vi "Assert DB Update Value.vi"() -> ()   [LabVIEW 2015, in "Database.lvclass"]
uses:
  Database.lvclass
panel:
  in  "table":string="钱凌峰ExcuseNote"
  in  "condition":string="Where 姓名= '钱凌峰' and 学号='1110810220' and 日期='2016/9/26' and 请假开始节次 = 2 and 请假结束节次 = 2"
  in  "path":path
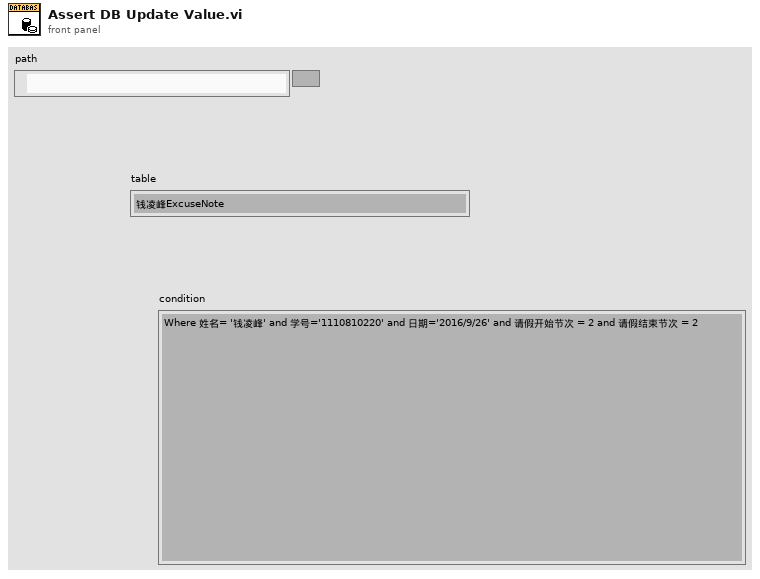
[diagram p1: front panel]
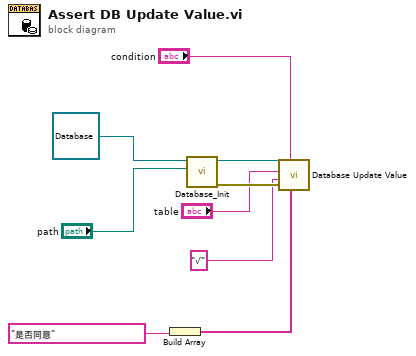
[diagram p0: block diagram]
diagram:
  n1 = Build Array("是否同意") -> (w2:string[])
  n2 = call "Database_Init.vi"("path"="path", "object in"=refnum<class "Database.lvclass"> refnum) -> ("error out"=w6:errorcluster, "object out"=w7:refnum<class "Database.lvclass">)  [unwired: 8 in]
  n3 = call "Database Update Value.vi"("columns"=w2, "condition"="condition", "error in (no error)"=w6, "data"="√", "table"="table", "Database in"=w7) -> ()  [unwired: 4 in, 2 out]
